vi "simple.vi"() -> ()   [LabVIEW 2018]
panel:
  out "Sum":dbl
  in  "A":dbl
  in  "B":dbl
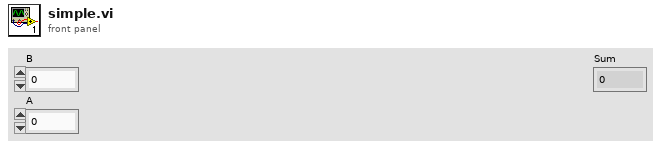
[diagram p1: front panel]
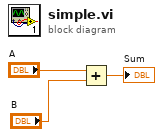
[diagram p0: block diagram]
diagram:
  n1 = Add(x="A", y="B") -> (x+y=→"Sum":dbl)
